vi "Log Status.vi"(8 "error in":errorcluster, 9 "Event Data String (-)":string="-", 10 "Event String":string, 11 "Log File Refnum In":refnum<file>) -> (0 "error out":errorcluster, 3 "Log File Refnum Out":refnum<file>)   [LabVIEW 2014]
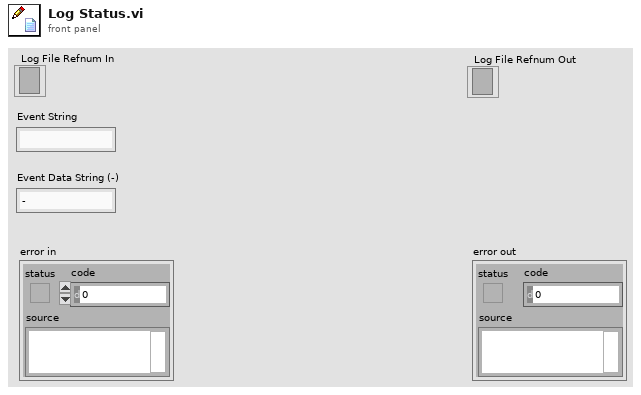
[diagram p1: front panel]
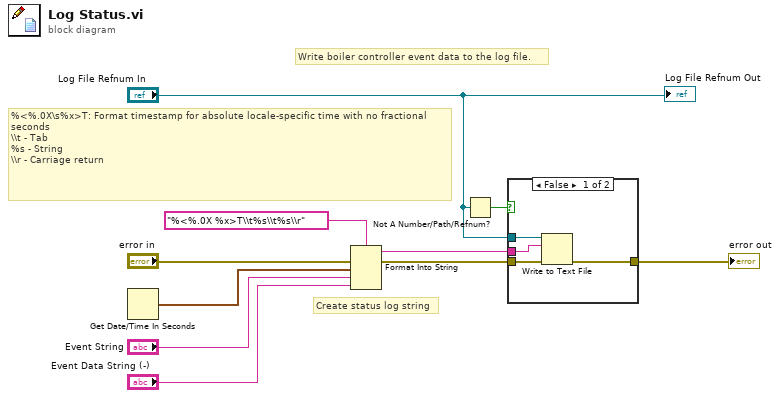
[diagram p0: block diagram]
diagram:
  # "%<%.0X\\s%x>T: Format timestamp for absolute locale-specific time with no fractional seconds\n\\\\t - Tab\n%s - String\n\\\\r - Carriage return"
  # "Create status log string"
  # "Write boiler controller event data to the log file."
  n1 = Get Date/Time In Seconds() -> (seconds since 1Jan1904=w8:timestamp)
  n2 = Format Into String(format string="%<%.0X %x>T\\t%s\\t%s\\r", error in="error in", w8, "Event String", "Event Data String (-)") -> (resulting string=w3:string, error out=w4:errorcluster)  [unwired: 1 in]
  n3 = Not A Number/Path/Refnum?(number/path/refnum="Log File Refnum In") -> (NaN/Path/Refnum?=w9:bool)
  n4 = case shown="False" w9 {
    tunnel: [w14 w15] -> w10
    tunnel: w3 -> [w13 _]
    tunnel: w4 -> [w12 w15]
    tunnel: "Log File Refnum In" -> [w11 _]
    frame False {
      n5 = Write to Text File(file (use dialog)=w11, text=w13, error in=w12) -> (error out=w14:errorcluster)  [unwired: 1 in, 2 out]
    }
    frame True {
    }
  }
  "error out" <- w10
  "Log File Refnum Out" <- "Log File Refnum In"
